vi "InitAppState.vi"   [LabVIEW 2013]
uses:
  GlobalVariables/AppState.vi
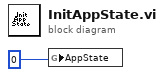
[diagram p0: block diagram]
diagram:
  n1 = global write "AppState.vi" "AppState"(u16 0 ("MachineState")) -> ()
